vi "EnQ Helper Loop Q DVR.vi"(9 "Helper Loop":refnum<class "Helper Loop.lvclass">, 10 "Helper Loop Q DVR":refnum<data-value>) -> (0 "error out":errorcluster)   [LabVIEW 2021, in "Helper Loop.lvclass"]
uses:
  Helper Loop.lvclass
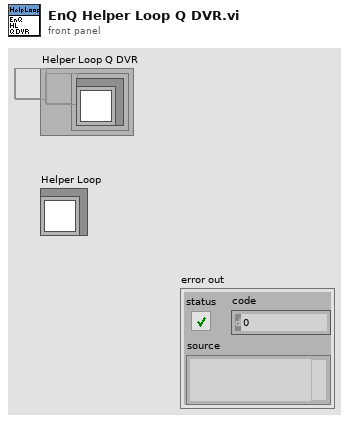
[diagram p1: front panel]
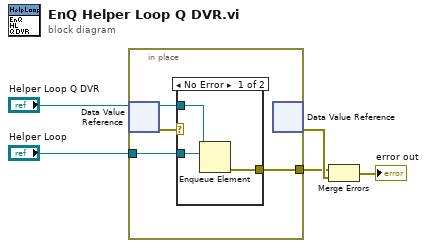
[diagram p0: block diagram]
diagram:
  n1 = in-place {
    in-place-border: "Helper Loop" -> [w9]
    in-place-border: [w8] -> w4
    n2 = in-place-dvr #1("Helper Loop Q DVR") -> (w7:refnum<queue>, w6:errorcluster)
    n3 = case shown="No Error" w6 {
      selector: w6 -> [_ w13]
      tunnel: w9 -> [w12 _]
      tunnel: [w11 w13] -> w8
      tunnel: w7 -> [w10 _]
      frame No Error {
        n4 = Enqueue Element(queue=w10, element=w12) -> (error out=w11:errorcluster)  [unwired: 2 in, 2 out]
      }
      frame Error {
      }
    }
    n5 = in-place-dvr #1() -> (w5:errorcluster)  [unwired: 1 in, 1 out]
  }
  n6 = Merge Errors(w4, w5) -> (→"error out":errorcluster)
